vi "Close.vi"(8 "error in (no error)":errorcluster caption="entrée d'erreur (pas d'erreur)", 11 "Class Spectrum_Analyser RS306B en entrée":refnum<class "Class Spectrum_Analyser RS306B.lvclass">) -> (0 "error out":errorcluster caption="sortie d'erreur", 3 "Class Spectrum_Analyser RS306B en sortie":refnum<class "Class Spectrum_Analyser RS306B.lvclass">)   [LabVIEW 2020, in "Library Instrument & Equipement.lvlib" / "Library Spectrum Analyser.lvlib" / "Class Spectrum_Analyser RS306B.lvclass"]
uses:
  Class Spectrum_Analyser RS306B.lvclass
  C:/Users/ngarcin/OneDrive - Altyor/Standard TB/Class/Spectrum Analyser/Class Spectrum Analyser (Default)/Class Spectrum Analyser (Default).lvclass
  Class Spectrum_Analyser RS306B.lvclass/Class Spectrum_Analyser RS306B.ctl
  Library Spectrum Analyser.lvlib
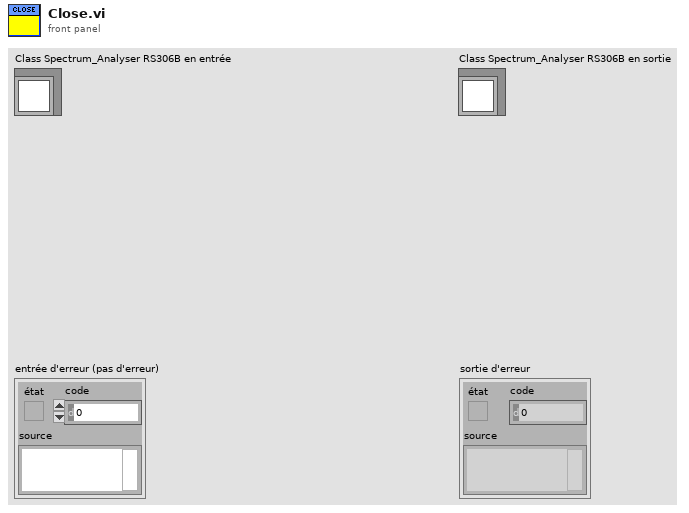
[diagram p1: front panel]
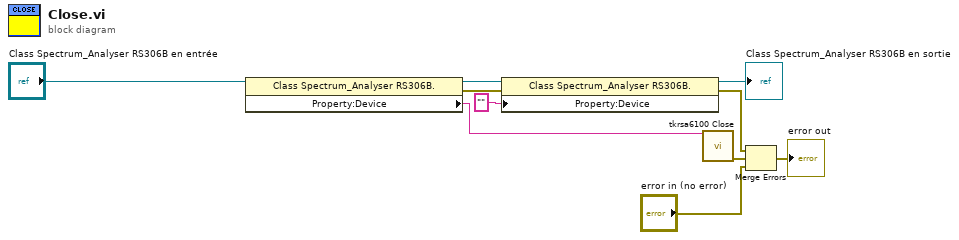
[diagram p0: block diagram]
diagram:
  n1 = property class="Class Spectrum_Analyser RS306B."(reference="Class Spectrum_Analyser RS306B en entrée") -> (reference out=w5:refnum<class "Class Spectrum_Analyser RS306B.lvclass">, error out=w2:errorcluster, "Property:Device"=w6:string)  [unwired: 1 in]
  n2 = property class="Class Spectrum_Analyser RS306B."(reference=w5, error in=w2, "Property:Device"="" ("Device")) -> (reference out=→"Class Spectrum_Analyser RS306B en sortie":refnum<class "Class Spectrum_Analyser RS306B.lvclass">, error out=w1:errorcluster)
  n3 = call "tkrsa6100 Close.vi"("VISA Resource Name"=w6) -> ("error out"=w10:errorcluster)  [unwired: 14 in]
  n4 = Merge Errors(w1, w10, "error in (no error)") -> (→"error out":errorcluster)
